vi "11-1.vi"() -> ()   [LabVIEW 2019, in "11.lvlib"]
uses:
  11.lvlib
panel:
  out "Flashes":u64
  out "Octo":i16[][](array[ring])
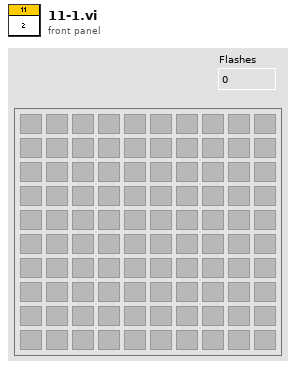
[diagram p1: front panel]
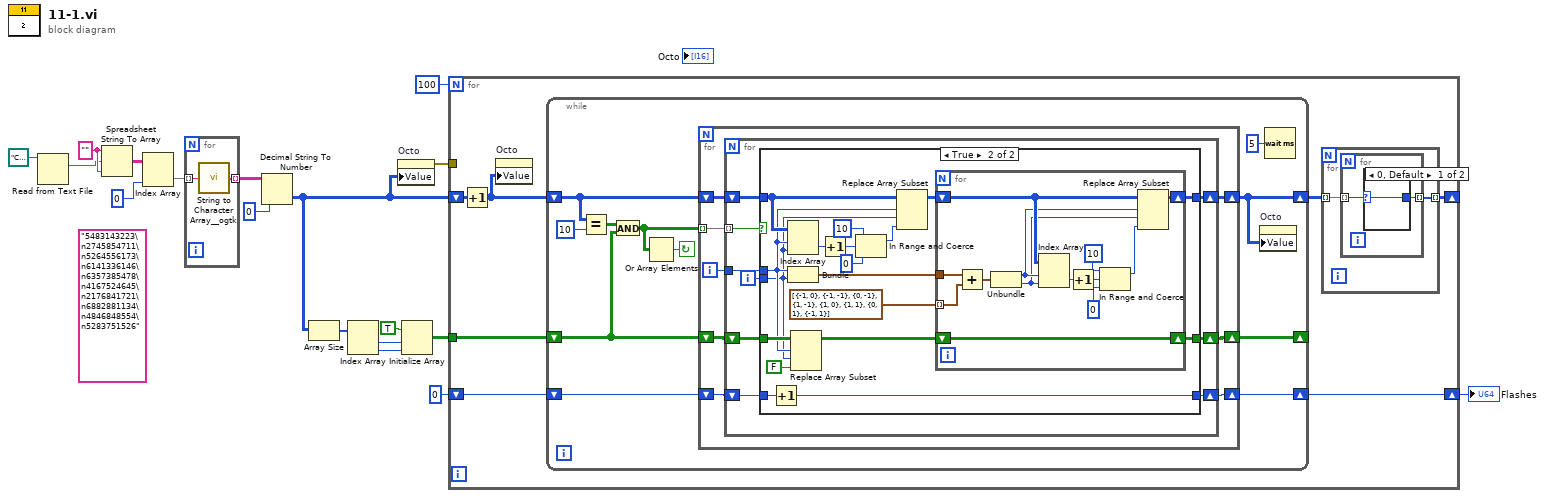
[diagram p0: block diagram]
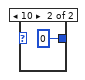
[diagram p3: hidden frame]
diagram:
  w18 = "" ("format string")
  (unwired) "5483143223\n2745854711\n5264556173\n6141336146\n6357385478\n4167524645\n2176841721\n6882881134\n4846848554\n5283751526"
  n1 = Read from Text File(file (use dialog)=path "C:/Users/craig.walker/Documents/GitHub/lv2019-Advent-of-Code-2021/11/input.txt") -> (text=w2:string)  [unwired: 3 in, 3 out]
  n2 = Spreadsheet String To Array(format string=w18, spreadsheet string=w2, array type (2D Dbl)=w18) -> (array=w17:string[][])  [unwired: 1 in]
  n3 = Index Array(array=w17, index (col)=0 ("disabled index (col)")) -> (element=w15:string[])  [unwired: 1 in]
  n4 = for {
    tunnel: w15 -> [w20] mode=indexing
    tunnel: [w19] -> w14 mode=indexing
    n5 = call <userlib>:"String to Character Array__ogtk.vi"("Input String"=w20) -> ("Character Array"=w19:string[])
  }
  n6 = Decimal String To Number(string=w14, default (0L)=i16 0 ("Octo")) -> (number=w11:i16[][])  [unwired: 1 in, 1 out]
  n7 = Array Size(array=w11) -> (size(s)=w10:i32[])
  n8 = Index Array(array=w10) -> (element #1=w9:i32, element #2=w8:i32)  [unwired: 2 in]
  n9 = property on="Octo" class="Arr (strict)"("Value"=w11) -> (error out=w12:errorcluster)  [unwired: 2 in, 1 out]
  n10 = Initialize Array(TRUE, w9, w8) -> (w6:bool[][])
  n11 = for {
    N: 100 -> [_]
    tunnel: w12 -> [_]
    shift-right: [w24] -> _
    shift-left: w11 -> [w27]
    tunnel: w6 -> [w25]
    shift-right: [w22] -> w4
    shift-left: u64 0 -> [w23]
    n12 = Increment(x=w27) -> (x+1=w26:i16[][])
    n13 = property on="Octo" class="Arr (strict)"("Value"=w26) -> ()  [unwired: 2 in, 2 out]
    n14 = while {
      shift-right: [w35] -> w21
      shift-left: w26 -> [w38]
      shift-right: [w31] -> _
      shift-left: w25 -> [w32]
      shift-right: [w29] -> w22
      shift-left: w23 -> [w30]
      stop <- w36 continue-if-true
      n15 = Equal?(x=w38, y=i16 10) -> (x = y?=w34:bool[][])
      n16 = And(x=w34, y=w32) -> (x .and. y?=w33:bool[][])
      n17 = Or Array Elements(Boolean array=w33) -> (logical OR=w36:bool)
      n18 = for {
        tunnel: w33 -> [w46] mode=indexing
        shift-right: [w43] -> w35
        shift-left: w38 -> [w45]
        shift-right: [w41] -> w31
        shift-left: w32 -> [w42]
        shift-right: [w39] -> w29
        shift-left: w30 -> [w40]
        i -> [w44]
        n19 = for {
          tunnel: w46 -> [w55] mode=indexing
          tunnel: w44 -> [w53]
          shift-right: [w51] -> w43
          shift-left: w45 -> [w54]
          shift-right: [w49] -> w41
          shift-left: w42 -> [w50]
          shift-right: [w47] -> w39
          shift-left: w40 -> [w48]
          i -> [w52]
          n20 = case shown="True" w55 {
            tunnel: w54 -> [w58 w74]
            tunnel: w53 -> [_ w70]
            tunnel: w52 -> [_ w69]
            tunnel: [w58 w62] -> w51
            tunnel: w50 -> [w57 w72]
            tunnel: [w57 w63] -> w49
            tunnel: w48 -> [w56 w61]
            tunnel: [w56 w60] -> w47
            frame False {
            }
            frame True {
              n21 = Increment(x=w61) -> (x+1=w60:u64)
              n22 = Index Array(array=w74, index (row)=w70, index (col)=w69) -> (element=w75:i16)
              n23 = Bundle(w70, w69) -> (w76:cluster{i32, i32})  [unwired: 1 in]
              n24 = Replace Array Subset(array=w72, new element=FALSE ("new element/subarray"), index (row)=w70, index (col)=w69) -> (w71:bool[][])
              n25 = Increment(x=w75) -> (x+1=w65:i16)
              n26 = In Range and Coerce(upper limit=i16 10, x=w65, lower limit=i16 0) -> (coerced(x)=w64:i16)  [unwired: 1 out]
              n27 = Replace Array Subset(array=w74, new element=w64, index (row)=w70, index (col)=w69) -> (w73:i16[][])
              n28 = for {
                tunnel: cluster{"Row":i32, "Col":i32}[] [{"Row"=-1, "Col"=0}, {"Row"=-1, "Col"=-1}, {"Row"=0, "Col"=-1}, {"Row"=1, "Col"=-1}, {"Row"=1, "Col"=0}, {"Row"=1, "Col"=1}, {"Row"=0, "Col"=1}, {"Row"=-1, "Col"=1}] -> [w88] mode=indexing
                tunnel: w76 -> [w89]
                shift-right: [w80] -> w62
                shift-left: w73 -> [w81]
                shift-right: [w77] -> w63
                shift-left: w71 -> [w77]
                n29 = Add(x=w89, y=w88) -> (x+y=w87:cluster{i32, i32})
                n30 = Unbundle(w87) -> (w79:i32, w78:i32)
                n31 = Index Array(array=w81, index (row)=w79, index (col)=w78) -> (element=w86:i16)
                n32 = Increment(x=w86) -> (x+1=w83:i16)
                n33 = In Range and Coerce(upper limit=i16 10, x=w83, lower limit=i16 0) -> (coerced(x)=w82:i16)  [unwired: 1 out]
                n34 = Replace Array Subset(array=w81, new element=w82, index (row)=w79, index (col)=w78) -> (w80:i16[][])
              }
            }
          }
        }
      }
      n35 = property on="Octo" class="Arr (strict)"("Value"=w35) -> ()  [unwired: 2 in, 2 out]
      n36 = Wait (ms)(milliseconds to wait=u32 5) -> ()  [unwired: 1 out]
    }
    n37 = for {
      tunnel: w21 -> [w91] mode=indexing
      tunnel: [w90] -> w24 mode=indexing
      n38 = for {
        tunnel: w91 -> [w93] mode=indexing
        tunnel: [w92] -> w90 mode=indexing
        n39 = case shown="0, Default" w93 {
          selector: w93 -> [w94 _]
          tunnel: [w94 i16 0 ("String")] -> w92
          frame 0, Default {
          }
          frame 10 {
          }
        }
      }
    }
  }
  "Flashes" <- w4
